vi "Control Type.vi"(11 "SequencedValves in":refnum<class "SeqDelayControl.lvclass">) -> (2 "Valve Type":string)   [LabVIEW 2020, in "VolatusControl.lvlib" / "SeqDelayControl.lvclass"]
uses:
  SeqDelayControl.lvclass
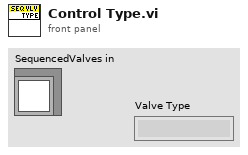
[diagram p1: front panel]
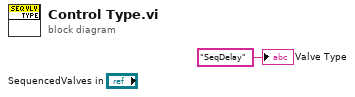
[diagram p0: block diagram]
diagram:
  "Valve Type" <- "SeqDelay" ("Valve Type")
